vi "Read Length-Prefixed String.vi"(0 "connection ID":refnum<k5>, 11 "error in (no error)":errorcluster) -> (4 "connection ID out":refnum<k5>, 8 "string":string, 15 "error out":errorcluster)   [LabVIEW 2020, in "epl-network.lvlib"]
uses:
  epl-network.lvlib
panel:
  in  "byte order":T1(ring)=enum."little-endian"
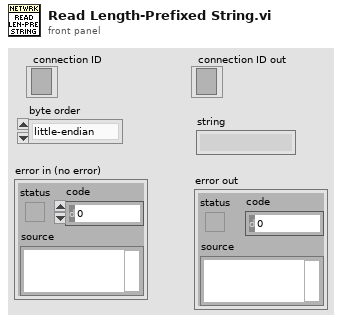
[diagram p1: front panel]
types:
  T1 = enum16{"big-endian, network order", "native, host order", "little-endian"}
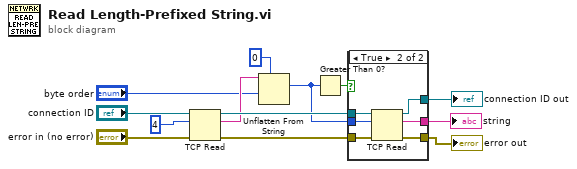
[diagram p0: block diagram]
diagram:
  n1 = TCP Read(connection ID="connection ID", bytes to read=4, error in (no error)="error in (no error)") -> (connection ID out=w10:refnum<k5>, data out=w5:string, error out=w9:errorcluster)  [unwired: 2 in]
  n2 = Unflatten From String(type=0, binary string=w5, byte order (0:big-endian, network order)="byte order") -> (value=w1:i32)  [unwired: 2 in, 2 out]
  n3 = Greater Than 0?(x=w1) -> (x > 0?=w8:bool)
  n4 = case shown="True" w8 {
    tunnel: [_ w21] -> w13
    tunnel: [w15 w20] -> w12
    tunnel: w10 -> [w14 w19]
    tunnel: w9 -> [w15 w18]
    tunnel: w1 -> [_ w17]
    tunnel: [w14 w16] -> w6
    frame False {
    }
    frame True {
      n5 = TCP Read(connection ID=w19, bytes to read=w17, error in (no error)=w18) -> (connection ID out=w16:refnum<k5>, data out=w21:string, error out=w20:errorcluster)  [unwired: 2 in]
    }
  }
  "string" <- w13
  "error out" <- w12
  "connection ID out" <- w6
